vi "Write Boolean.vi"(8 "error in (no error)":errorcluster, 10 "Boolean":bool, 11 "ZanCard in":refnum<class "ZanCard.lvclass">) -> (0 "error out":errorcluster, 3 "ZanCard out":refnum<class "ZanCard.lvclass">)   [LabVIEW 2019, in "ZanCard.lvclass"]
uses:
  ZanCard.lvclass
  ZanCard.lvclass/ZanCard.ctl
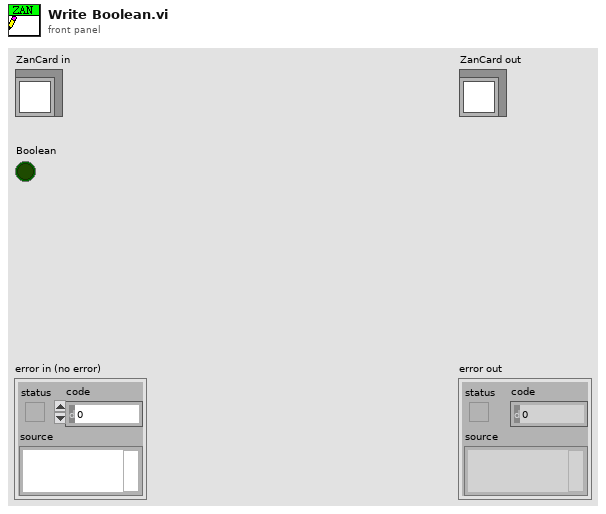
[diagram p1: front panel]
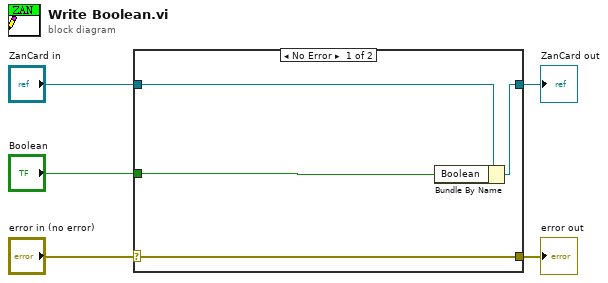
[diagram p0: block diagram]
diagram:
  n1 = case shown="No Error" "error in (no error)" {
    selector: "error in (no error)" -> [w9 w10]
    tunnel: [w9 w10] -> w4
    tunnel: [w7 w11] -> w2
    tunnel: "ZanCard in" -> [w8 w11]
    tunnel: "Boolean" -> [w6 _]
    frame No Error {
      n2 = Bundle By Name(cluster=w8, "Boolean"=w6) -> (w7:refnum<class "ZanCard.lvclass">)
    }
    frame Error {
    }
  }
  "error out" <- w4
  "ZanCard out" <- w2
